vi "Drive Get.vi"(1 "Y":dbl, 2 "Slow Drive":bool, 3 "X":dbl) -> ()   [LabVIEW 2013]
uses:
  Drive Global Data.vi
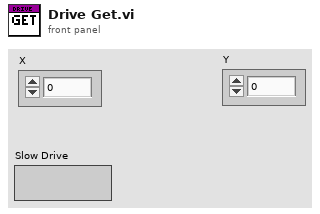
[diagram p1: front panel]
types:
  T1 = cluster{"Y":dbl, "X":dbl, "Left Encoder":dbl, "Right Encoder":dbl, "Slow Drive":bool}
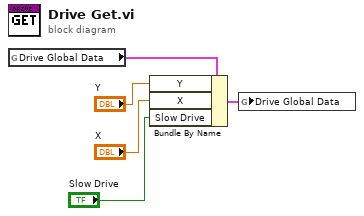
[diagram p0: block diagram]
diagram:
  n1 = global read "Drive Global Data.vi" "Drive Global Data"() -> (w5:T1)
  n2 = Bundle By Name(cluster=w5, "Y"="Y", "X"="X", "Slow Drive"="Slow Drive") -> (w2:T1)
  n3 = global write "Drive Global Data.vi" "Drive Global Data"(w2) -> ()
